vi "listRemoteDir.vi"(8 "error in (no error)":errorcluster, 9 "ConnectionData":T1, 10 "remote path":string, 11 "TreeControlRefIn":refnum<vi>) -> (0 "error out":errorcluster, 3 "TreeControlRefOut":refnum<vi>)   [LabVIEW 2015]
uses:
  General/RemoteFiles/connectionData.ctl
panel:
  # "Lists the contents of a remote directory via SSH, and populatea a tree control with it. \nThis uses the plink.exe utility to perform this.\nDOWNLOAD: http://www.chiark.greenend.org.uk/~sgtatham/putty/download.html"
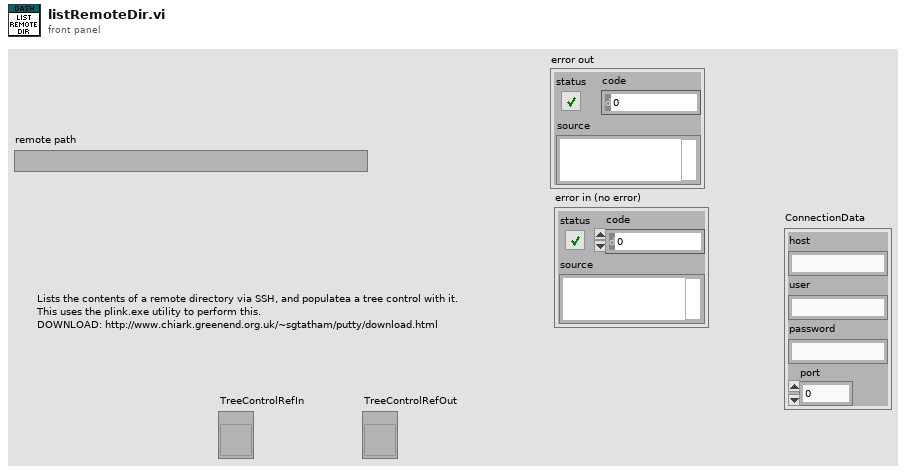
[diagram p1: front panel]
types:
  T1 = typedef "connectionData.ctl" = cluster{"host":string, "user":string, "password":string, "port":u16}
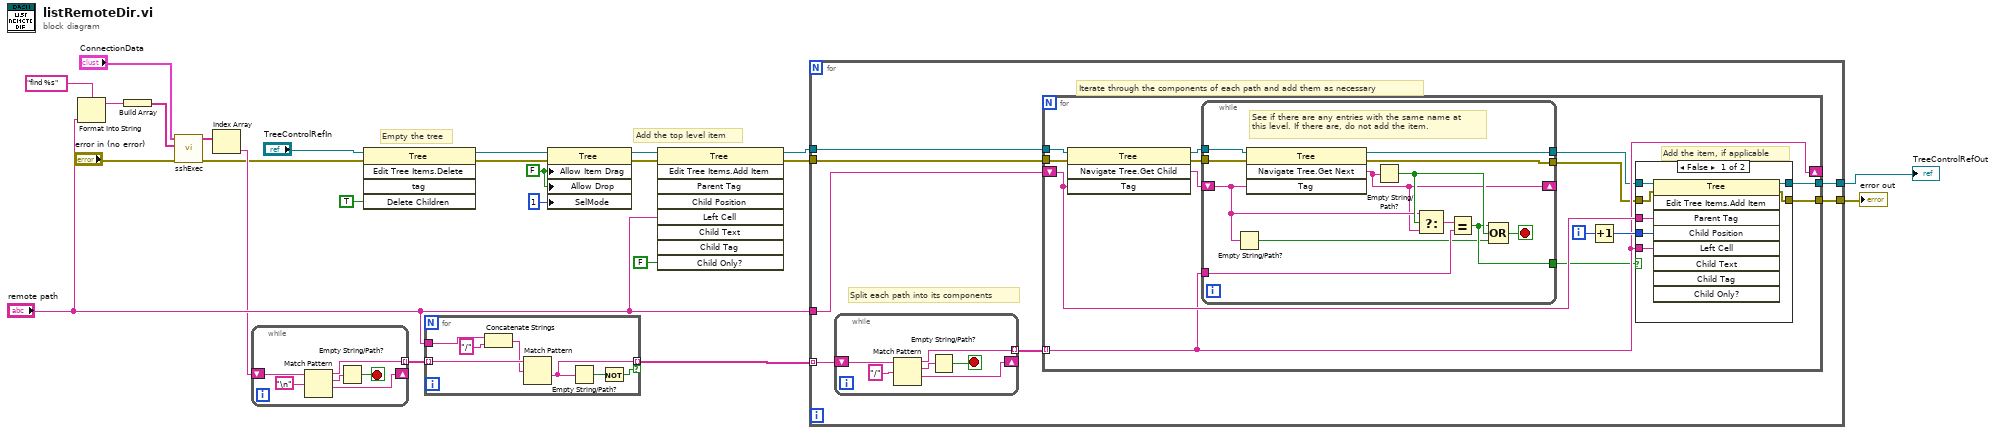
[diagram p0: block diagram]
diagram:
  w1 = FALSE ("Drag/Drop:Allow Dragging")
  # "Empty the tree"
  # "Add the top level item"
  n1 = Format Into String(format string="find %s", "remote path") -> (resulting string=w16:string)  [unwired: 2 in, 1 out]
  n2 = Build Array(w16) -> (w15:string[])
  n3 = call "sshExec.vi"("error in"="error in (no error)", "Commands"=w15, "ConnectionData"="ConnectionData") -> ("error out"=w11:errorcluster, "Output"=w14:string[])  [unwired: 7 in]
  n4 = Index Array(array=w14) -> (element=w13:string)  [unwired: 1 in]
  n5 = while {
    shift-right: [w28] -> _
    shift-left: w13 -> [w30]
    tunnel: [w27] -> w12 mode=indexing
    stop <- w25 stop-if-true
    n6 = Match Pattern(string=w30, regular expression="\n") -> (before substring=w27:string, match substring=w26:string, after substring=w28:string)  [unwired: 1 in, 1 out]
    n7 = Empty String/Path?(string/path=w26) -> (empty?=w25:bool)
  }
  n8 = invoke class="Tree" method="Edit Tree Items.Delete"(reference="TreeControlRefIn", error in=w11, "Delete Children"=TRUE ("Delete Children?")) -> (reference out=w6:refnum<vi>, error out=w5:errorcluster)  [unwired: 2 in, 3 out]
  n9 = for {
    tunnel: w12 -> [w37] mode=indexing
    tunnel: "remote path" -> [w36]
    tunnel: [w33] -> w23 mode=indexing if=w31
    n10 = Concatenate Strings(w36, "/" ("string")) -> (w35:string)
    n11 = Match Pattern(string=w37, regular expression=w35) -> (after substring=w33:string)  [unwired: 1 in, 3 out]
    n12 = Empty String/Path?(string/path=w33) -> (empty?=w32:bool)
    n13 = Not(x=w32) -> (.not. x?=w31:bool)
  }
  n14 = property class="Tree"(reference=w6, error in=w5, "Allow Item Drag"=w1, "Allow Drop"=w1, "SelMode"=1 ("Selection Mode")) -> (reference out=w4:refnum<vi>, error out=w3:errorcluster)
  n15 = invoke class="Tree" method="Edit Tree Items.Add Item"(reference=w4, error in=w3, "Left Cell"="remote path", "Child Only?"=FALSE) -> (reference out=w21:refnum<vi>, error out=w10:errorcluster)  [unwired: 5 in, 7 out]
  n16 = for {
    tunnel: w23 -> [w44] mode=indexing
    tunnel: w21 -> [w42]
    tunnel: "remote path" -> [w41]
    tunnel: [w40] -> w7
    tunnel: w10 -> [w39]
    tunnel: [w38] -> w9
    # "Iterate through the components of each path and add them as necessary"
    # "Split each path into its components"
    n17 = while {
      shift-right: [w84] -> _
      shift-left: w44 -> [w85]
      tunnel: [w83] -> w43 mode=indexing
      stop <- w81 stop-if-true
      n18 = Match Pattern(string=w85, regular expression="/") -> (before substring=w83:string, match substring=w82:string, after substring=w84:string)  [unwired: 1 in, 1 out]
      n19 = Empty String/Path?(string/path=w82) -> (empty?=w81:bool)
    }
    n20 = for {
      tunnel: w43 -> [w53] mode=indexing
      tunnel: w42 -> [w51]
      shift-right: [w53] -> _
      shift-left: w41 -> [w56]
      tunnel: [w46] -> w40
      tunnel: w39 -> [w49]
      tunnel: [w45] -> w38
      i -> [w58]
      # "Add the item, if applicable"
      n21 = invoke class="Tree" method="Navigate Tree.Get Child"(reference=w51, error in=w49, "Tag"=w56) -> (reference out=w54:refnum<vi>, error out=w48:errorcluster, "Navigate Tree:Get Child"=w55:string)  [unwired: 1 in, 1 out]
      n22 = while {
        tunnel: w54 -> [w70]
        tunnel: w53 -> [w68]
        tunnel: [w65] -> w52
        shift-right: [w62] -> _
        shift-left: w55 -> [w64]
        tunnel: [w61] -> w50
        tunnel: w48 -> [w60]
        tunnel: [w59] -> w47
        stop <- w67 stop-if-true
        # "See if there are any entries with the same name at\nthis level. If there are, do not add the item."
        n23 = Empty String/Path?(string/path=w64) -> (empty?=w63:bool)
        n24 = invoke class="Tree" method="Navigate Tree.Get Next"(reference=w70, error in=w60, "Tag"=w64) -> (reference out=w61:refnum<vi>, error out=w59:errorcluster, "Navigate Tree:Get Next Item"=w62:string)  [unwired: 1 in, 1 out]
        n25 = Empty String/Path?(string/path=w62) -> (empty?=w66:bool)
        n26 = Select(t=w64, s=w66, f=w62) -> (s? t:f=w69:string)
        n27 = Equal?(x=w69, y=w68) -> (x = y?=w65:bool)
        n28 = Compound Arithmetic op=OR(w65, w66, w63) -> (w67:bool)
      }
      n29 = Increment(x=w58) -> (x+1=w57:i32)
      n30 = case shown="False" w52 {
        tunnel: w56 -> [w77 _]
        tunnel: w57 -> [w76 _]
        tunnel: w53 -> [w75 _]
        tunnel: w50 -> [w74 w79]
        tunnel: w47 -> [w73 w78]
        tunnel: [w72 w79] -> w46
        tunnel: [w71 w78] -> w45
        frame False {
          n31 = invoke class="Tree" method="Edit Tree Items.Add Item"(reference=w74, error in=w73, "Parent Tag"=w77, "Child Position"=w76, "Left Cell"=w75) -> (reference out=w72:refnum<vi>, error out=w71:errorcluster)  [unwired: 4 in, 7 out]
        }
        frame True {
        }
      }
    }
  }
  "TreeControlRefOut" <- w7
  "error out" <- w9
